vi "Write Record Data.vi"(8 "Error In (no error)":errorcluster, 10 "Record":variant, 11 "Expenses Tracker Cycle In":refnum<class "Expenses Tracker Cycle.lvclass">) -> (0 "Error Out":errorcluster, 3 "Expenses Tracker Cycle Out":refnum<class "Expenses Tracker Cycle.lvclass">)   [LabVIEW 2023, in "Expenses Tracker Cycle.lvclass"]
uses:
  Expenses Tracker Cycle.lvclass
  Ctrls/Cycle.ctl
  Expenses Tracker Cycle.lvclass/Expenses Tracker Cycle.ctl
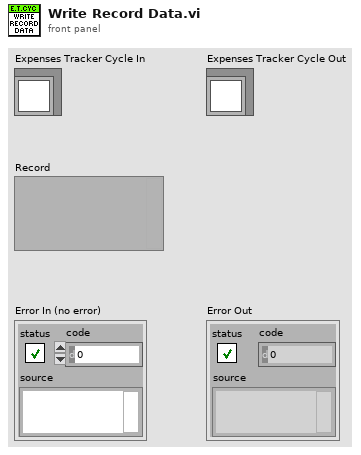
[diagram p1: front panel]
types:
  T1 = typedef "Expenses Tracker Cycle.lvclass/Cycle.ctl" = cluster{"ID":u32, "Name":string, "Day_of_occurence":u8, "Description":string}
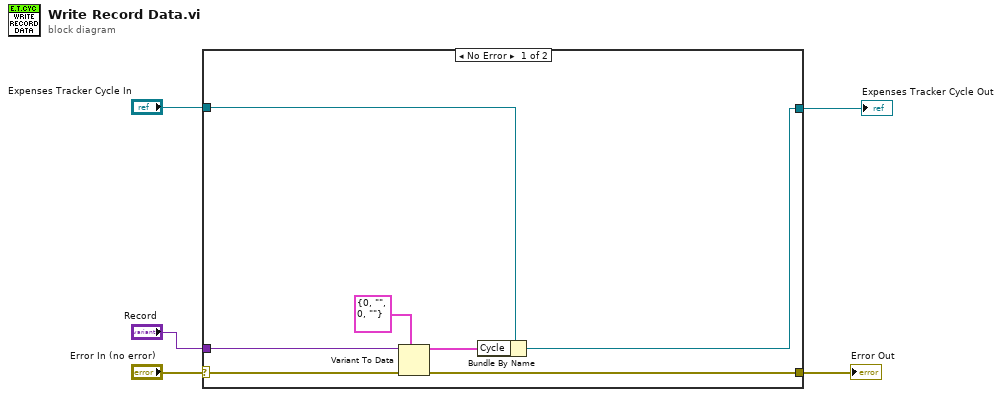
[diagram p0: block diagram]
diagram:
  n1 = case shown="No Error" "Error In (no error)" {
    selector: "Error In (no error)" -> [w10 w14]
    tunnel: [w8 w14] -> w4
    tunnel: [w7 w13] -> w3
    tunnel: "Expenses Tracker Cycle In" -> [w6 w13]
    tunnel: "Record" -> [w12 _]
    frame No Error {
      n2 = Variant To Data(error in=w10, type=T1 {"ID"=0, "Name"="", "Day_of_occurence"=0, "Description"=""} ("Cycle"), Variant=w12) -> (data=w11:T1, error out=w8:errorcluster)
      n3 = Bundle By Name(cluster=w6, "Cycle"=w11) -> (w7:refnum<class "Expenses Tracker Cycle.lvclass">)
    }
    frame Error {
    }
  }
  "Error Out" <- w4
  "Expenses Tracker Cycle Out" <- w3
